vi "ExtendedRegisterWrite.vi"(7 "Extended Read/Write":T1 {"Data" format="%.0x"; "Register" format="%.0x"; "Slave Address" max=15 format="%.0x"}, 8 "error in (no error)":errorcluster, 9 "Number of Samples In":i32, 10 "Data Array":u8[][](array[numeric]), 11 "RFFE_Data In":T2 {"Toggle (high to low)" items=["0", "1", "Z", "L", "H", "X", "T", "V"]; "X Array" items=["0", "1", "Z", "L", "H", "X", "T", "V"]; "Z Array" items=["0", "1", "Z", "L", "H", "X", "T", "V"]; "L Array" items=["0", "1", "Z", "L", "H", "X", "T", "V"]; "H Array" items=["0", "1", "Z", "L", "H", "X", "T", "V"]; "One Array" items=["0", "1", "Z", "L", "H", "X", "T", "V"]; "Zero Array" items=["0", "1", "Z", "L", "H", "X", "T", "V"]}) -> (0 "error out":errorcluster, 1 "Number of Samples Out":i32, 2 "Data Array Out":u8[][](array[numeric]), 3 "RFFE_Data Out":T2 {"Toggle (high to low)" items=["0", "1", "Z", "L", "H", "X", "T", "V"]; "X Array" items=["0", "1", "Z", "L", "H", "X", "T", "V"]; "Z Array" items=["0", "1", "Z", "L", "H", "X", "T", "V"]; "L Array" items=["0", "1", "Z", "L", "H", "X", "T", "V"]; "H Array" items=["0", "1", "Z", "L", "H", "X", "T", "V"]; "One Array" items=["0", "1", "Z", "L", "H", "X", "T", "V"]; "Zero Array" items=["0", "1", "Z", "L", "H", "X", "T", "V"]})   [LabVIEW 2013]
doc: "Builds MIPI RFFE Extended Register Write with the specified data."
uses:
  Ctrls/RFFE_Data.ctl
  Ctrls/ClockDataChannels.ctl
  Ctrls/ExtendedRegReadWrite.ctl
  Ctrls/Commands.ctl
  Ctrls/Read_Write_Data.ctl
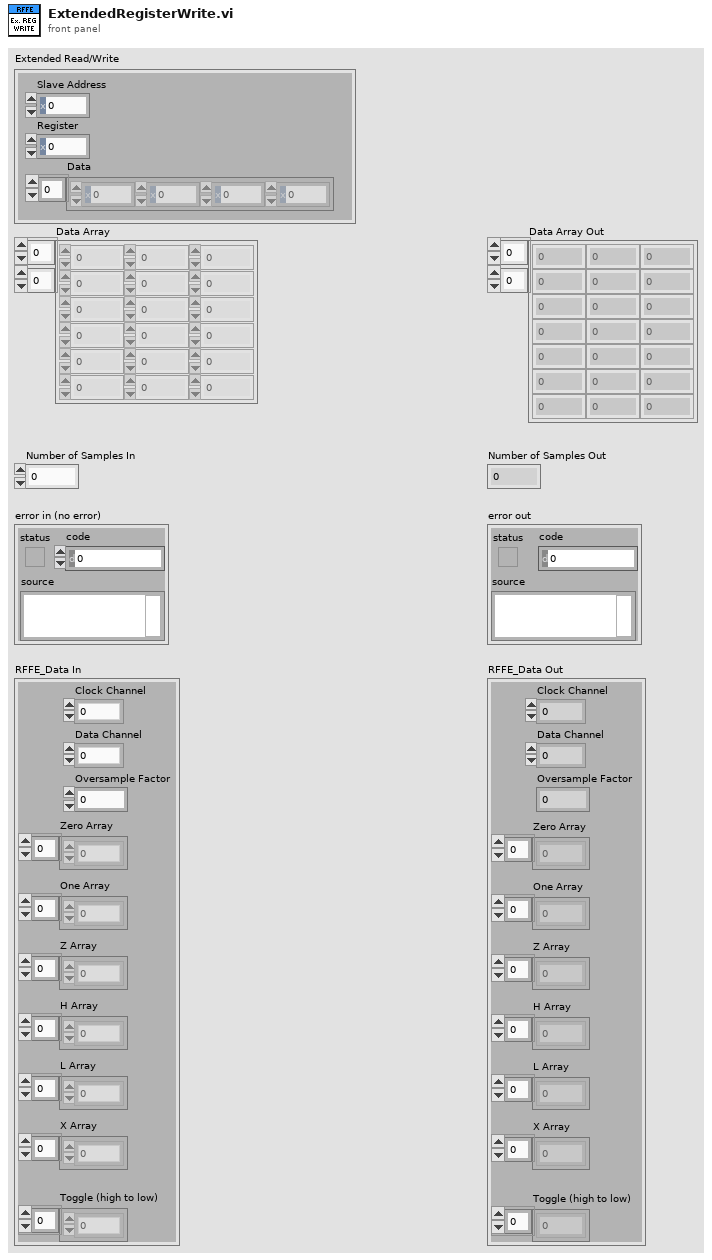
[diagram p1: front panel]
types:
  T1 = typedef "ExtendedRegReadWrite.ctl" = cluster{"Slave Address":u8, "Register":u8, "Data":u8[]}
  T2 = typedef "RFFE_Data.ctl" = cluster{"Clock Channel":T3, "Data Channel":T3, "Oversample Factor":u8, "Zero Array":u8[], "One Array":u8[], "Z Array ":u8[], "H Array":u8[], "L Array":u8[], "X Array":u8[], "Toggle (high to low)":u8[]}
  T3 = typedef "ClockDataChannels.ctl" = enum16{"0", "1"}
  T4 = typedef "Read_Write_Data.ctl" = cluster{"Data":u8, "Read/Write":enum16{"Read", "Write"}}
  T5 = typedef "Commands.ctl" = cluster{"Command":enum16{"Extended Register Write", "Extended Register Read", "Extended Register Write Long", "Extended Register Read Long", "Register Write", "Register Read", "Register 0 Write"}, "Data/Address/ByteCount":u8}
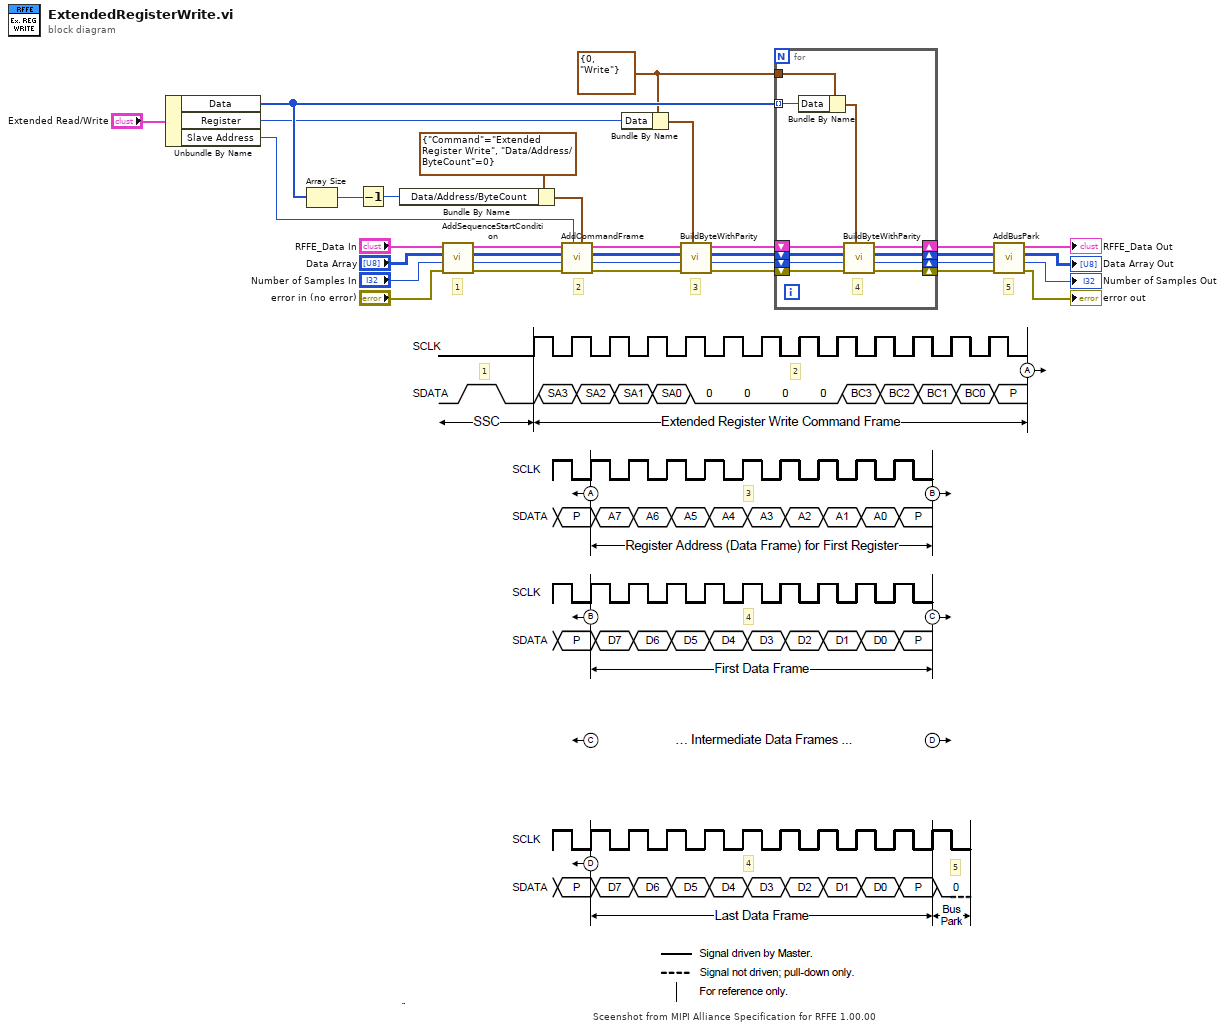
[diagram p0: block diagram]
diagram:
  w14 = T4 {"Data"=0, "Read/Write"=enum."Write"} ("Read/Write Data")
  # "Sceenshot from MIPI Alliance Specification for RFFE 1.00.00"
  # "4"
  # "5"
  # "4"
  # "3"
  # "2"
  # "1"
  # "5"
  # "3"
  # "2"
  # "1"
  n1 = Unbundle By Name("Extended Read/Write") -> ("Data"=w15:u8[], "Register"=w8:u8, "Slave Address"=w1:u8)
  n2 = Array Size(array=w15) -> (size(s)=w16:i32)
  n3 = Decrement(x=w16) -> (x-1=w3:i32)
  n4 = Bundle By Name(cluster=T5 {"Command"=enum."Extended Register Write", "Data/Address/ByteCount"=0} ("Command"), "Data/Address/ByteCount"=w3) -> (w2:T5)
  n5 = call "AddSequenceStartCondition.vi"("error in (no error)"="error in (no error)", "Number of Samples In"="Number of Samples In", "Data Array In"="Data Array", "RFFE_Data In"="RFFE_Data In") -> ("error out"=w28:errorcluster, "Number of Samples Out"=w32:i32, "Data Array Out"=w29:u8[][], "RFFE_Data Out"=w30:T2)  [unwired: 4 in]
  n6 = call "AddCommandFrame.vi"("Command"=w2, "Slave Address"=w1, "error in (no error)"=w28, "Number of Samples In"=w32, "Data Array In"=w29, "RFFE_Data"=w30) -> ("error out"=w6:errorcluster, "Number of Samples Out"=w5:i32, "Data Array Out"=w4:u8[][], "Configuratation Out"=w7:T2)  [unwired: 2 in]
  n7 = Bundle By Name(cluster=w14, "Data"=w8) -> (w9:T4)
  n8 = call "BuildByteWithParity.vi"("Read/Write Data"=w9, "error in"=w6, "Number of Samples In"=w5, "Data Array In"=w4, "RFFE_Data In"=w7) -> ("error out"=w13:errorcluster, "Number of Samples Out"=w12:i32, "Data Array Out"=w11:u8[][], "RFFE_Data Out"=w10:T2)  [unwired: 2 in, 1 out]
  n9 = for {
    shift-right: [w44] -> w20
    shift-left: w13 -> [w45]
    shift-right: [w41] -> w17
    shift-left: w12 -> [w43]
    shift-right: [w40] -> w18
    shift-left: w11 -> [w42]
    shift-right: [w39] -> w19
    shift-left: w10 -> [w38]
    tunnel: w15 -> [w37] mode=indexing
    tunnel: w14 -> [w35]
    # "4"
    n10 = Bundle By Name(cluster=w35, "Data"=w37) -> (w36:T4)
    n11 = call "BuildByteWithParity.vi"("Read/Write Data"=w36, "error in"=w45, "Number of Samples In"=w43, "Data Array In"=w42, "RFFE_Data In"=w38) -> ("error out"=w44:errorcluster, "Number of Samples Out"=w41:i32, "Data Array Out"=w40:u8[][], "RFFE_Data Out"=w39:T2)  [unwired: 2 in, 1 out]
  }
  n12 = call "AddBusPark.vi"("error in (no error)"=w20, "Number of Samples In"=w17, "Data Array In"=w18, "RFFE_Data In"=w19) -> ("error out"=→"error out":errorcluster, "Number of Samples Out"=→"Number of Samples Out":i32, "Data Array Out"=→"Data Array Out":u8[][], "RFFE_Data Out"=→"RFFE_Data Out":T2)  [unwired: 4 in]
